vi "Bind To Type.vi"(8 "error in (no error)":errorcluster, 10 "Type Name":string, 11 "Malicious Serialization Binder in":refnum<class "Malicious Serialization Binder.lvclass">) -> (0 "error out":errorcluster, 2 "Type":refnum<class>, 3 "Malicious Serialization Binder out":refnum<class "Malicious Serialization Binder.lvclass">)   [LabVIEW 2017, in "Generic Object Serializer Tests.lvlib" / "Malicious Serialization Binder.lvclass"]
doc: "Controls the binding of a serialized object to a type."
uses:
  Malicious Serialization Binder.lvclass
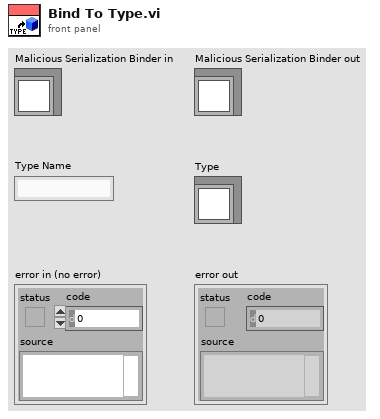
[diagram p1: front panel]
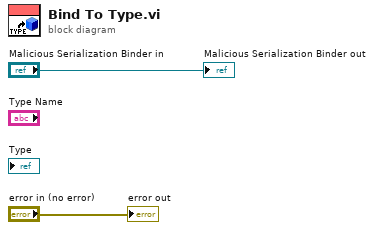
[diagram p0: block diagram]
diagram:
  "error out" <- "error in (no error)"
  "Malicious Serialization Binder out" <- "Malicious Serialization Binder in"
